vi "PH_Beckhoff-16BB.contents.vi"   [LabVIEW 2014, in "PH_Beckhoff-16BB.lvlib"]
doc: "This class is forseen to xxx\n\nThis class is part of the PHELIX xxx layer."
uses:
  PH_Beckhoff-16BB.lvlib
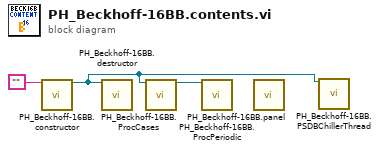
[diagram p0: block diagram]
diagram:
  n1 = call "PH_Beckhoff-16BB.constructor.vi"("name"="") -> ("i ref out"=w1:refnum<vi>)  [unwired: 16 in, 2 out]
  n2 = call "PH_Beckhoff-16BB.destructor.vi"("i ref in"=w1) -> ()  [unwired: 18 in, 1 out]
  n3 = call "PH_Beckhoff-16BB.ProcCases.vi"("i ref in"=w1) -> ("i ref out"=w2:refnum<vi>)  [unwired: 16 in, 2 out]
  n4 = call "PH_Beckhoff-16BB.ProcPeriodic.vi"("i ref in"=w2) -> ()  [unwired: 16 in, 3 out]
  n5 = call "PH_Beckhoff-16BB.panel.vi"() -> ()  [unwired: 19 in, 1 out]
  n6 = call "PH_Beckhoff-16BB.PSDBChillerThread.vi"("object ref"=w1) -> ()  [unwired: 18 in, 1 out]
